vi "Kill Process.vi"(8 "error in (no error)":errorcluster, 11 "process name":string="softioc.exe") -> (0 "error out":errorcluster, 1 "standard error":string, 3 "process name out":string="NITaggerService", 4 "console out":string="SERVICE_NAME: NITaggerService\r\nTRUE")   [LabVIEW 2017]
doc: "Terminates the Windows process named by str and returns its standard error and console output."
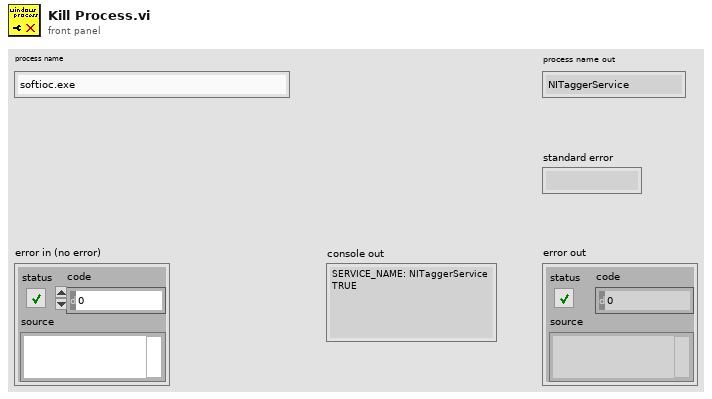
[diagram p1: front panel]
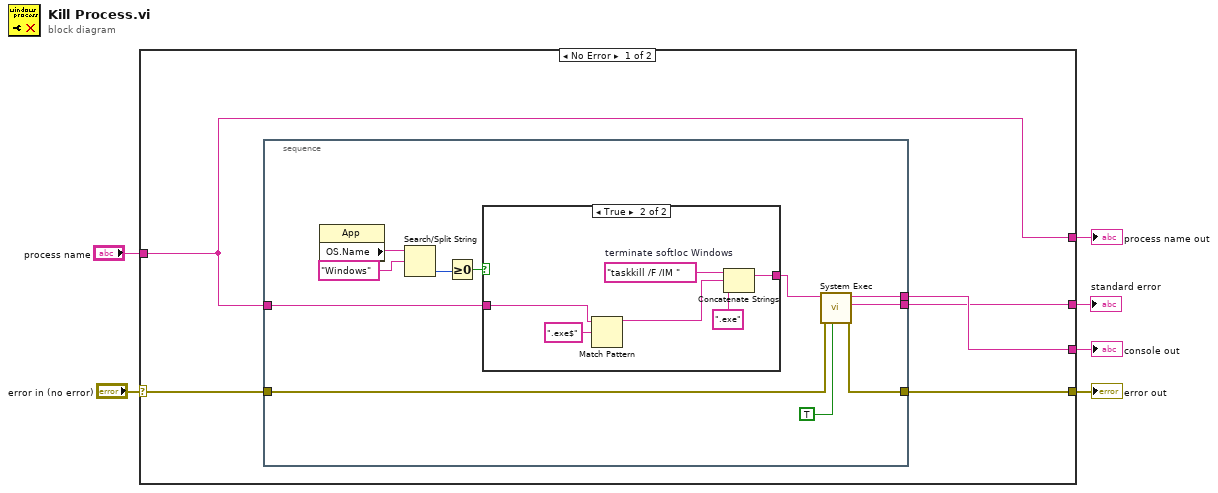
[diagram p0: block diagram]
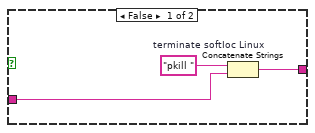
[diagram p2: hidden frame]
diagram:
  n1 = case shown="No Error" "error in (no error)" {
    selector: "error in (no error)" -> [w8 w32]
    tunnel: [w11 _] -> w6
    tunnel: "process name" -> [w11 _]
    tunnel: [w10 _] -> w4
    tunnel: [w9 w32] -> w2
    tunnel: [w7 _] -> w1
    frame No Error {
      n2 = stacked-sequence {
        tunnel: [w17] -> w9
        tunnel: [w16] -> w7
        tunnel: [w15] -> w10
        tunnel: w11 -> [w22]
        tunnel: w8 -> [w12]
        frame #0 {
          n3 = property class="App"() -> ("OS.Name"=w18:string)  [unwired: 2 in, 2 out]
          n4 = Search/Split String(string=w18, search string/char (-)="Windows" ("Operating System:Name")) -> (offset of match=w19:i32)  [unwired: 3 out]
          n5 = Greater Or Equal To 0?(x=w19) -> (x >= 0?=w21:bool)
          n6 = case shown="True" w21 {
            tunnel: [w23 w29] -> w14
            tunnel: w22 -> [w24 w28]
            frame False {
              w25 = "pkill "  # terminate softIoc Linux
              n7 = Concatenate Strings(w25, w24) -> (w23:string)
            }
            frame True {
              w30 = "taskkill /F /IM "  # terminate softIoc Windows
              n8 = Match Pattern(string=w28, regular expression=".exe$") -> (before substring=w26:string)  [unwired: 1 in, 3 out]
              n9 = Concatenate Strings(w30, w26, ".exe" ("string")) -> (w29:string)
            }
          }
          n10 = call <vilib>:"System Exec.vi"("run minimized? (F)"=TRUE, "error in (no error)"=w12, "command line"=w14) -> ("error out"=w17:errorcluster, "standard error"=w16:string, "standard output"=w15:string)  [unwired: 3 in, 3 out]
        }
      }
    }
    frame Error {
    }
  }
  "console out" <- w4
  "process name out" <- w6
  "error out" <- w2
  "standard error" <- w1
